vi "Restart.vi"(8 "error in (no error)":errorcluster) -> ()   [LabVIEW 2015]
uses:
  <vilib>/nisyscfg/Close (System).vi
  <vilib>/nisyscfg/nisyscfg.lvlib
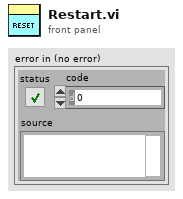
[diagram p1: front panel]
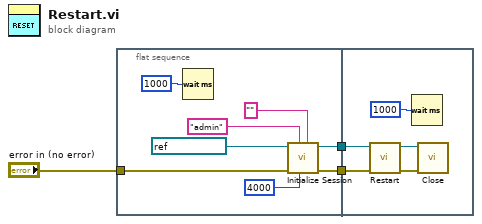
[diagram p0: block diagram]
diagram:
  n1 = flat-sequence {
    tunnel: [w6] -> w3
    tunnel: [w5] -> w2
    tunnel: "error in (no error)" -> [w4]
    tunnel: w3 -> [w15]
    tunnel: w2 -> [w12]
    frame #0 {
      n2 = Wait (ms)(milliseconds to wait=u32 1000) -> ()  [unwired: 1 out]
      n3 = call <vilib>:"Initialize Session.vi"("Password"="", "Connect Timeout (4000 ms)"=u32 4000, "User Name"="admin", "error in (no error)"=w4, "Target (localhost)"=refnum<k21> "localhost") -> ("error out"=w5:errorcluster, "Session out"=w6:refnum<k21>)  [unwired: 5 in]
    }
    frame #1 {
      n4 = call <vilib>:"Restart.vi"("error in (no error)"=w12, "Session in"=w15) -> ("error out"=w13:errorcluster, "Session out"=w14:refnum<k21>)  [unwired: 7 in, 1 out]
      n5 = Wait (ms)(milliseconds to wait=u32 1000) -> ()  [unwired: 1 out]
      n6 = call-poly <vilib>:"Close.vi"("error in (no error)"=w13, "Session in"=w14) -> ()  [unwired: 9 in, 1 out]
    }
  }
